vi "ShutDownSubVI.vi"(1 "shutdown":bool) -> (0 "Shut Down":u32)   [LabVIEW 2017]
uses:
  atmcd32d.dll
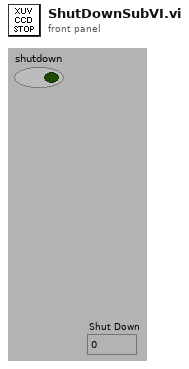
[diagram p1: front panel]
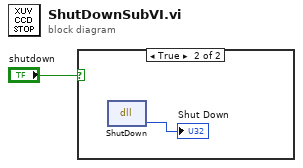
[diagram p0: block diagram]
diagram:
  n1 = case shown="True" "shutdown" {
    frame False {
    }
    frame True {
      n2 = dll-call lib="atmcd32d.dll" fn="ShutDown" label="Call Library Function Shutdown"() -> (→"Shut Down":u32)  [unwired: 3 in, 2 out]
    }
  }
